vi "tm_getparameter_40.vi"(6 "Index":i32, 7 "Reconfigure (F)":bool, 8 "error in (no error)":errorcluster, 10 "Parameter":u32(ring)=4215968 items=["SENSOR MODE"=4212128, "SENSOR MODE LINE BUNDLE HEIGHT"=4212192, "READOUT DIRECTION"=4211904, "BIT PER CHANNEL"=4342976, "EXPOSURE TIME"=2049184, "CONTRAST GAIN"=3163312, "BINNING"=4215968, "TIMING READOUT TIME"=4223904, "INTERNAL FRAME RATE"=4225952, "INTERNAL FRAME INTERVAL"=4225968, "INTERNAL LINE SPEED"=4226000, "IMAGE WIDTH"=4343200, "IMAGE HEIGHT"=4343216, "IMAGE ROWBYTES"=4343232, "IMAGE FRAMEBYTES"=4343248, "IMAGE PIXEL TYPE"=4343296], 11 "Handle in":u32) -> (0 "error out":errorcluster, 2 "Value out":dbl, 3 "Handle out":u32)   [LabVIEW 2023]
uses:
  tmcamcon.dll
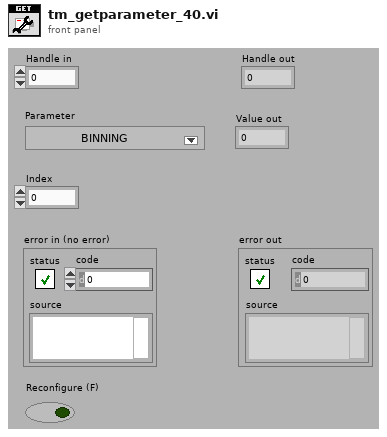
[diagram p1: front panel]
types:
  T1 = cluster{"Property Name":string, "Property ID":i32}[]
  T2 = cluster{"Property Name":string, "Property ID":i32}
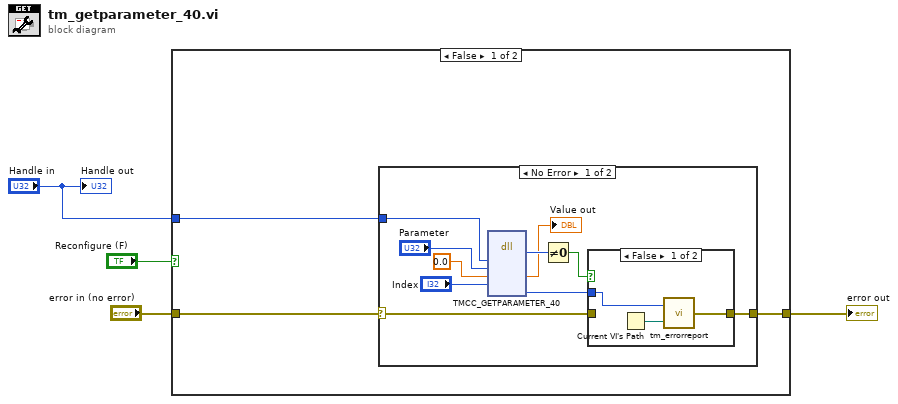
[diagram p0: block diagram]
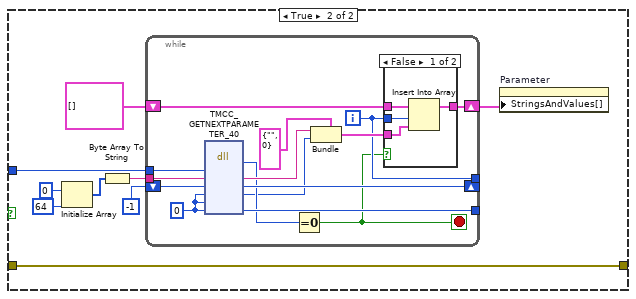
[diagram p4: hidden frame]
diagram:
  n1 = case shown="False" "Reconfigure (F)" {
    tunnel: "error in (no error)" -> [w6 w31]
    tunnel: [w7 w31] -> w3
    tunnel: "Handle in" -> [w5 w23]
    frame False {
      n2 = case shown="No Error" w6 {
        selector: w6 -> [w12 w22]
        tunnel: [w9 w22] -> w7
        tunnel: w5 -> [w16 _]
        frame No Error {
          n3 = dll-call lib="tmcamcon.dll" fn="TMCC_GETPARAMETER_40"("handle"=w16, "parameter"="Parameter", "value"=0.0, "view"="Index") -> ("return type"=w17:u32, "value"=→"Value out":dbl, "Erval"=w11:i32)  [unwired: 7 in, 2 out]
          n4 = Not Equal To 0?(x=w17) -> (x != 0?=w10:bool)
          n5 = case shown="False" w10 {
            tunnel: w12 -> [_ w21]
            tunnel: [w19 w21] -> w9
            tunnel: w11 -> [w18 _]
            frame False {
              n6 = Current VI's Path() -> (path=w20:path)
              n7 = call "tm_errorreport.vi"("Source"=w20, "Error"=w18) -> ("error out"=w19:errorcluster)
            }
            frame True {
            }
          }
        }
        frame Error {
        }
      }
    }
    frame True {
      n8 = Initialize Array(u8 0 ("element"), 64 ("dimension size")) -> (w26:u8[])
      n9 = Byte Array To String(unsigned byte array=w26) -> (string=w29:string)
      n10 = while {
        shift-right: [w45] -> w24
        shift-left: T1 [] ("Array") -> [w46]
        tunnel: [w41] -> _
        tunnel: [w39] -> _
        tunnel: w29 -> [w38]
        tunnel: w23 -> [w37]
        shift-right: [w40] -> _
        shift-left: -1 ("func_num") -> [w42]
        i -> [w39]
        stop <- w35 stop-if-true
        w32 = 0 ("option")
        n11 = dll-call lib="tmcamcon.dll" fn="TMCC_GETNEXTPARAMETER_40"("HDCAM"=w37, "name"=w38, "func_num"=w42, "func_id"=w32, "option"=w32, "Erval"=w32) -> ("return type"=w34:u32, "name"=w43:string, "func_num"=w40:i32, "func_id"=w33:i32, "Erval"=w41:i32)  [unwired: 5 in, 2 out]
        n12 = Equal To 0?(x=w34) -> (x = 0?=w35:bool)
        n13 = Bundle(cluster=T2 {"Property Name"="", "Property ID"=0} ("new element/subarray"), "Property Name"=w43, "Property ID"=w33) -> (w44:T2)
        n14 = case shown="False" w35 {
          tunnel: w46 -> [w50 w51]
          tunnel: [w49 w51] -> w45
          tunnel: w39 -> [w48 _]
          tunnel: w44 -> [w47 _]
          frame False {
            n15 = Insert Into Array(array=w50, index=w48, new element=w47) -> (w49:T1)
          }
          frame True {
          }
        }
      }
      n16 = property on="Parameter" class="Ring (strict)"("StringsAndValues[]"=w24) -> ()  [unwired: 2 in, 2 out]
    }
  }
  "error out" <- w3
  "Handle out" <- "Handle in"
